vi "Update Time Remaining Indicator.vi"(8 "error in (no error)":errorcluster, 10 "Time Remaining":dbl, 11 "Wash Display Console API in":refnum<class "Wash Display Console API.lvclass">) -> (0 "error out":errorcluster, 3 "Wash Display Console API out":refnum<class "Wash Display Console API.lvclass">)   [LabVIEW 2012, in "Wash Display Console API.lvlib" / "Wash Display Console API.lvclass"]
uses:
  Wash Display Console API.lvclass
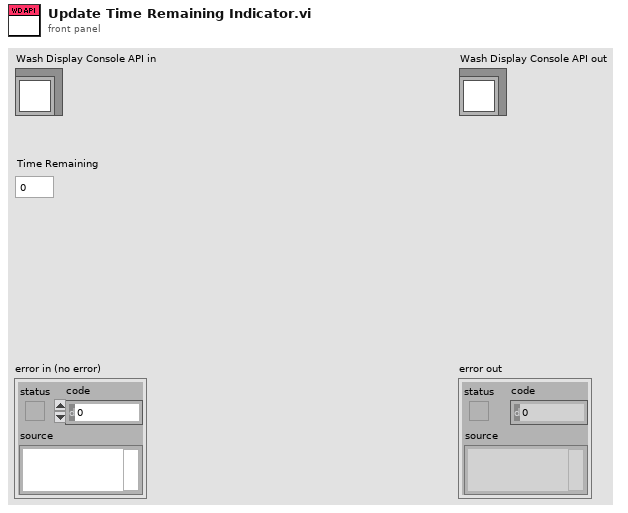
[diagram p1: front panel]
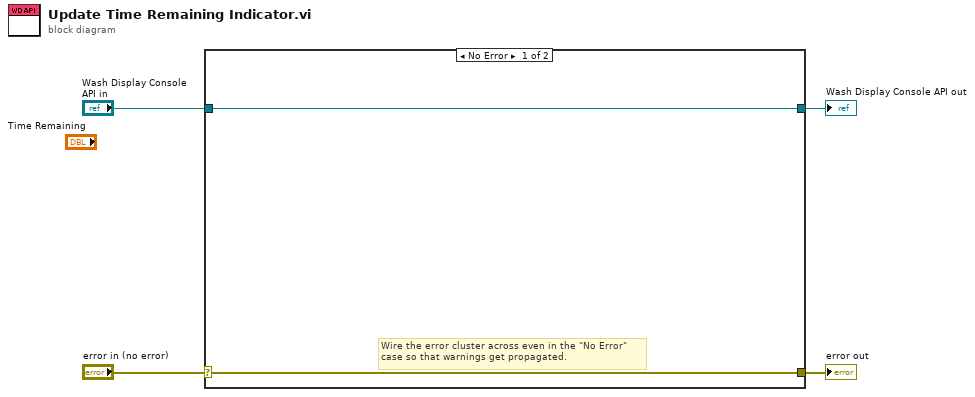
[diagram p0: block diagram]
diagram:
  n1 = case shown="No Error" "error in (no error)" {
    selector: "error in (no error)" -> [w5 w8]
    tunnel: [w5 w8] -> w3
    tunnel: [w6 w7] -> w1
    tunnel: "Wash Display Console API in" -> [w6 w7]
    frame No Error {
      # "Wire the error cluster across even in the \"No Error\"\ncase so that warnings get propagated."
    }
    frame Error {
    }
  }
  "error out" <- w3
  "Wash Display Console API out" <- w1
